vi "Write Jitter(px).vi"(8 "error in (no error)":errorcluster, 10 "Jitter(px)":u32, 11 "Camera Simulator in":refnum<class "Camera Simulator.lvclass">) -> (0 "error out":errorcluster, 3 "Camera Simulator out":refnum<class "Camera Simulator.lvclass">)   [LabVIEW 2020, in "Camera Simulator.lvlib" / "Camera Simulator.lvclass"]
uses:
  Camera Simulator.lvclass
  Camera Simulator.lvclass/Camera Simulator.ctl
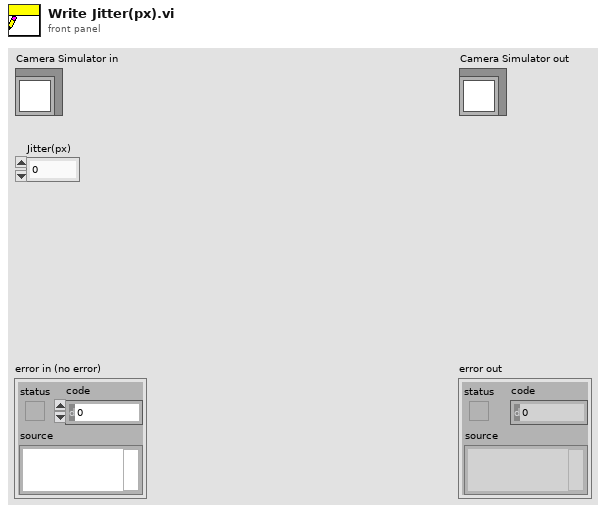
[diagram p1: front panel]
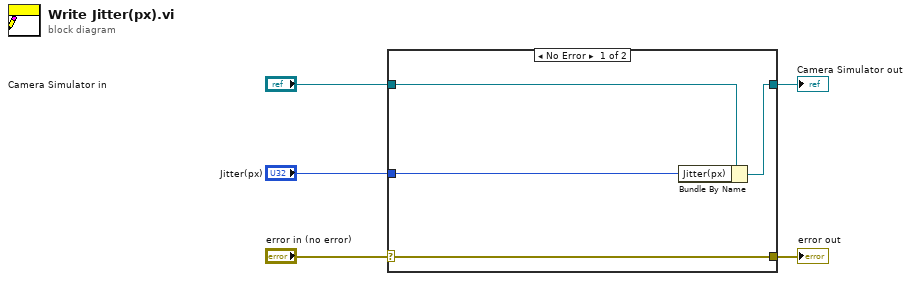
[diagram p0: block diagram]
diagram:
  n1 = case shown="No Error" "error in (no error)" {
    selector: "error in (no error)" -> [w9 w10]
    tunnel: [w9 w10] -> w4
    tunnel: [w7 w11] -> w2
    tunnel: "Camera Simulator in" -> [w8 w11]
    tunnel: "Jitter(px)" -> [w6 _]
    frame No Error {
      n2 = Bundle By Name(cluster=w8, "Jitter(px)"=w6) -> (w7:refnum<class "Camera Simulator.lvclass">)
    }
    frame Error {
    }
  }
  "error out" <- w4
  "Camera Simulator out" <- w2
